vi "DriveAuto.vi"   [LabVIEW 2015]
types:
  T1 = typedef "WPI_EncoderDevRef.ctl" = cluster{"DevStatus":errorcluster, "EncoderIndex":T2, "CounterIndex":T3, "DistancePerCount":dbl, "Decoding Type":T4}
  T2 = typedef "FPGA_EncoderIdx.ctl" = enum8{"Enc 0", "Enc 1", "Enc 2", "Enc 3", "Enc 4", "Enc 5", "Enc 6", "Enc 7", "Invalid"}
  T3 = typedef "FPGA_CounterCtrSystemIndex.ctl" = enum8{"Ctr 0", "Ctr 1", "Ctr 2", "Ctr 3", "Ctr 4", "Ctr 5", "Ctr 6", "Ctr 7", "Invalid"}
  T4 = typedef "WPI_EncoderType.ctl" = enum16{"1x", "2x", "4x"}
  T5 = typedef "WPI_MotorControlDeviceRef.ctl" = cluster{"DeviceStatus":errorcluster, "Type":T6, "PWM":cluster{"PWM Channel":T7, "DeadBand":T8}, "CAN":cluster{"Device Number":u8, "Control Mode":T9, "Semaphore":T10, "Max Vout":dbl, "TalonSRX Control Mode":T11}, "Invert":bool}
  T6 = typedef "WPI_MotorControlType.ctl" = enum16{"PWM", "CAN", "CANTalonSRX"}
  T7 = typedef "FPGA_DIOPWMChannel.ctl" = enum8{"PWM 0", "PWM 1", "PWM 2", "PWM 3", "PWM 4", "PWM 5", "PWM 6", "PWM 7", "PWM 8", "PWM 9", "PWM MXP 0", "PWM MXP 1", "PWM MXP 2", "PWM MXP 3", "PWM MXP 4", "PWM MXP 5", "PWM MXP 6", "PWM MXP 7", "PWM MXP 8", "PWM MXP 9", "Invalid"}
  T8 = typedef "WPI_PWMDeadband.ctl" = cluster{"Name":string, "maxPositivePwm":i32, "minPositivePwm":i32, "centerPwm":i32, "maxNegativePwm":i32, "minNegativePwm":i32, "angularRange":u16}
  T9 = typedef "WPI_CANJaguar_ControlMode.ctl" = enum8{"Percent VBus", "Current", "Speed", "Position", "Voltage"}
  T10 = typedef "Semaphore RefNum" = refnum<k1>
  T11 = typedef "WPI_CANTalonSRX_APIControlMode.ctl" = enum8{"Percent VBus", "Speed", "Position", "Slave", "Unchanged / Invalid", "Voltage Compensation", "Current", "Motion Profile"}
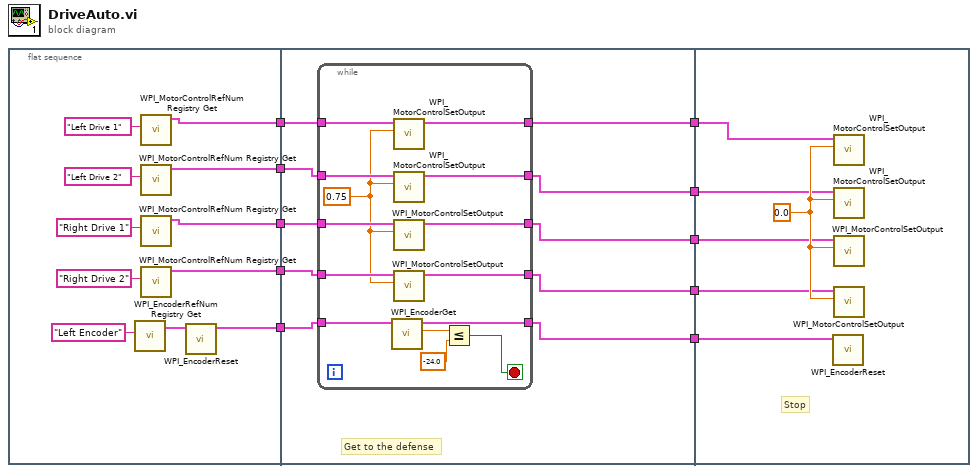
[diagram p0: block diagram]
diagram:
  n1 = flat-sequence {
    tunnel: [w11] -> w5
    tunnel: [w16] -> w4
    tunnel: [w15] -> w3
    tunnel: [w14] -> w2
    tunnel: [w13] -> w1
    tunnel: [w31] -> w10
    tunnel: [w30] -> w9
    tunnel: [w29] -> w8
    tunnel: [w28] -> w7
    tunnel: [w27] -> w6
    tunnel: w5 -> [w26]
    tunnel: w4 -> [w25]
    tunnel: w3 -> [w24]
    tunnel: w2 -> [w23]
    tunnel: w1 -> [w22]
    tunnel: w10 -> [w50]
    tunnel: w9 -> [w49]
    tunnel: w8 -> [w48]
    tunnel: w7 -> [w47]
    tunnel: w6 -> [w46]
    frame #0 {
      n2 = call <vilib>:"WPI_EncoderRefNum Registry Get.vi"("refnum name"="Left Encoder") -> ("EncoderDevRef"=w12:T1)  [unwired: 9 in, 1 out]
      n3 = call <vilib>:"WPI_MotorControlRefNum Registry Get.vi"("refnum name"="Left Drive 1") -> ("MotorControlDevRef"=w13:T5)  [unwired: 9 in, 1 out]
      n4 = call <vilib>:"WPI_MotorControlRefNum Registry Get.vi"("refnum name"="Left Drive 2") -> ("MotorControlDevRef"=w14:T5)  [unwired: 9 in, 1 out]
      n5 = call <vilib>:"WPI_MotorControlRefNum Registry Get.vi"("refnum name"="Right Drive 1") -> ("MotorControlDevRef"=w15:T5)  [unwired: 9 in, 1 out]
      n6 = call <vilib>:"WPI_MotorControlRefNum Registry Get.vi"("refnum name"="Right Drive 2") -> ("MotorControlDevRef"=w16:T5)  [unwired: 9 in, 1 out]
      n7 = call <vilib>:"WPI_EncoderReset.vi"("EncoderDevRef"=w12) -> ("EncoderDevRef"=w11:T1)  [unwired: 9 in, 1 out]
    }
    frame #1 {
      # "Get to the defense"
      n8 = while {
        tunnel: w22 -> [w45]
        tunnel: w23 -> [w44]
        tunnel: w24 -> [w43]
        tunnel: w25 -> [w42]
        tunnel: w26 -> [w40]
        tunnel: [w36] -> w31
        tunnel: [w35] -> w30
        tunnel: [w34] -> w29
        tunnel: [w33] -> w28
        tunnel: [w32] -> w27
        stop <- w38 stop-if-true
        w41 = 0.75 ("Output")
        n9 = call <vilib>:"WPI_EncoderGet.vi"("EncoderDevRef"=w40) -> ("Distance"=w39:dbl, "EncoderDevRef"=w32:T1)  [unwired: 5 in, 4 out]
        n10 = call <vilib>:"WPI_MotorControlSetOutput.vi"("Output"=w41, "MotorControlDevRef"=w45) -> ("MotorControlDevRef"=w36:T5)  [unwired: 7 in, 2 out]
        n11 = call <vilib>:"WPI_MotorControlSetOutput.vi"("Output"=w41, "MotorControlDevRef"=w44) -> ("MotorControlDevRef"=w35:T5)  [unwired: 7 in, 2 out]
        n12 = call <vilib>:"WPI_MotorControlSetOutput.vi"("Output"=w41, "MotorControlDevRef"=w43) -> ("MotorControlDevRef"=w34:T5)  [unwired: 7 in, 2 out]
        n13 = call <vilib>:"WPI_MotorControlSetOutput.vi"("Output"=w41, "MotorControlDevRef"=w42) -> ("MotorControlDevRef"=w33:T5)  [unwired: 7 in, 2 out]
        n14 = Less Or Equal?(x=w39, y=-24.0) -> (x <= y?=w38:bool)
      }
    }
    frame #2 {
      w51 = 0.0 ("Output")
      # "Stop"
      n15 = call <vilib>:"WPI_EncoderReset.vi"("EncoderDevRef"=w46) -> ()  [unwired: 9 in, 2 out]
      n16 = call <vilib>:"WPI_MotorControlSetOutput.vi"("Output"=w51, "MotorControlDevRef"=w50) -> ()  [unwired: 7 in, 3 out]
      n17 = call <vilib>:"WPI_MotorControlSetOutput.vi"("Output"=w51, "MotorControlDevRef"=w49) -> ()  [unwired: 7 in, 3 out]
      n18 = call <vilib>:"WPI_MotorControlSetOutput.vi"("Output"=w51, "MotorControlDevRef"=w48) -> ()  [unwired: 7 in, 3 out]
      n19 = call <vilib>:"WPI_MotorControlSetOutput.vi"("Output"=w51, "MotorControlDevRef"=w47) -> ()  [unwired: 7 in, 3 out]
    }
  }
